vi "Actor Core.vi"(8 "error in":errorcluster, 11 "Panel Helper in":refnum<class "Panel Helper.lvclass">) -> (0 "error out":errorcluster, 3 "Actor out":refnum<class "Actor.lvclass">)   [LabVIEW 2020, in "2. Basic Panel Actors.lvlib" / "Panel Helper.lvclass"]
doc: "The user interface for this panel.\n----\nCopyright: MGI 2016\nAuthor: Derek Trepanier"
uses:
  Panel Helper.lvclass
  C:/Program Files/National Instruments/LabVIEW 2020/vi.lib/MGI/Panel Manager/Panel Actor/Panel Actor/Panel Actor.lvclass
  <vilib>/ActorFramework/Actor/Actor.lvclass
  <vilib>/ActorFramework/Message Enqueuer/Message Enqueuer.lvclass/Message Enqueuer.ctl
  <vilib>/MGI/Panel Manager/Panel/Panel Helper/Panel Helper.lvclass/Panel Helper.ctl
  <vilib>/ActorFramework/Message Enqueuer/Enqueue.vi
  Description Panel/Description Panel.lvclass
  <vilib>/MGI/Panel Manager/Panel/Panel/Subpanel/Subpanel.lvclass
  C:/Program Files/National Instruments/LabVIEW 2020/vi.lib/MGI/Panel Manager/Panel/Panel/Panel.lvclass
  <vilib>/ActorFramework/Stop Msg/Stop Msg.lvclass
  C:/Program Files/National Instruments/LabVIEW 2020/vi.lib/ActorFramework/Message/Message.lvclass
  <vilib>/MGI/Panel Manager/Panel/Panel/Subpanel/Subpanel.vi
  <vilib>/ActorFramework/Message Priority Queue/Priority Enqueue.vi
  <vilib>/MGI/Panel Manager/Panel/Deferer/Deferer.lvclass
  <vilib>/MGI/Panel Manager/Panel Actor/Panel Actor/Panel Actor.lvclass
  <vilib>/MGI/Panel Manager/Panel/Panel Updater/Panel Updater.lvclass
  <vilib>/MGI/Panel Manager/Panel/Panel.lvlib
  <vilib>/MGI/Panel Manager/Panel/Panel Helper/Panel Helper.lvclass
panel:
  in  "Clear Title":bool
  in  "Panel Title Override":string
  in  "Clear Tree":bool
  in  "Without Defer":bool
  in  "With Defer":bool
  in  "Tree":string(tree)
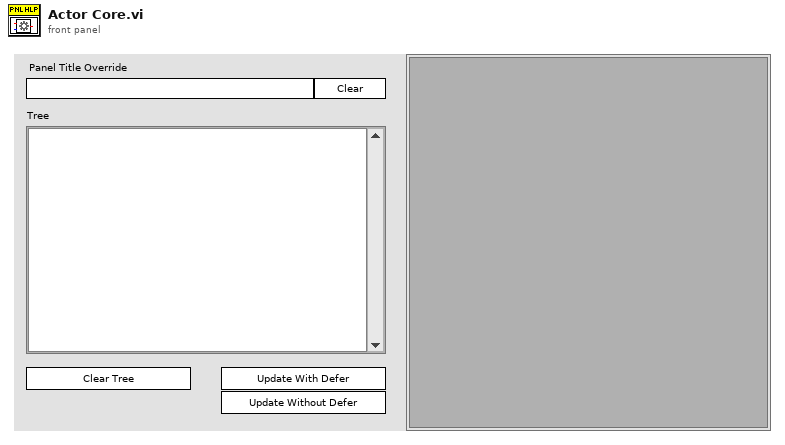
[diagram p1: front panel]
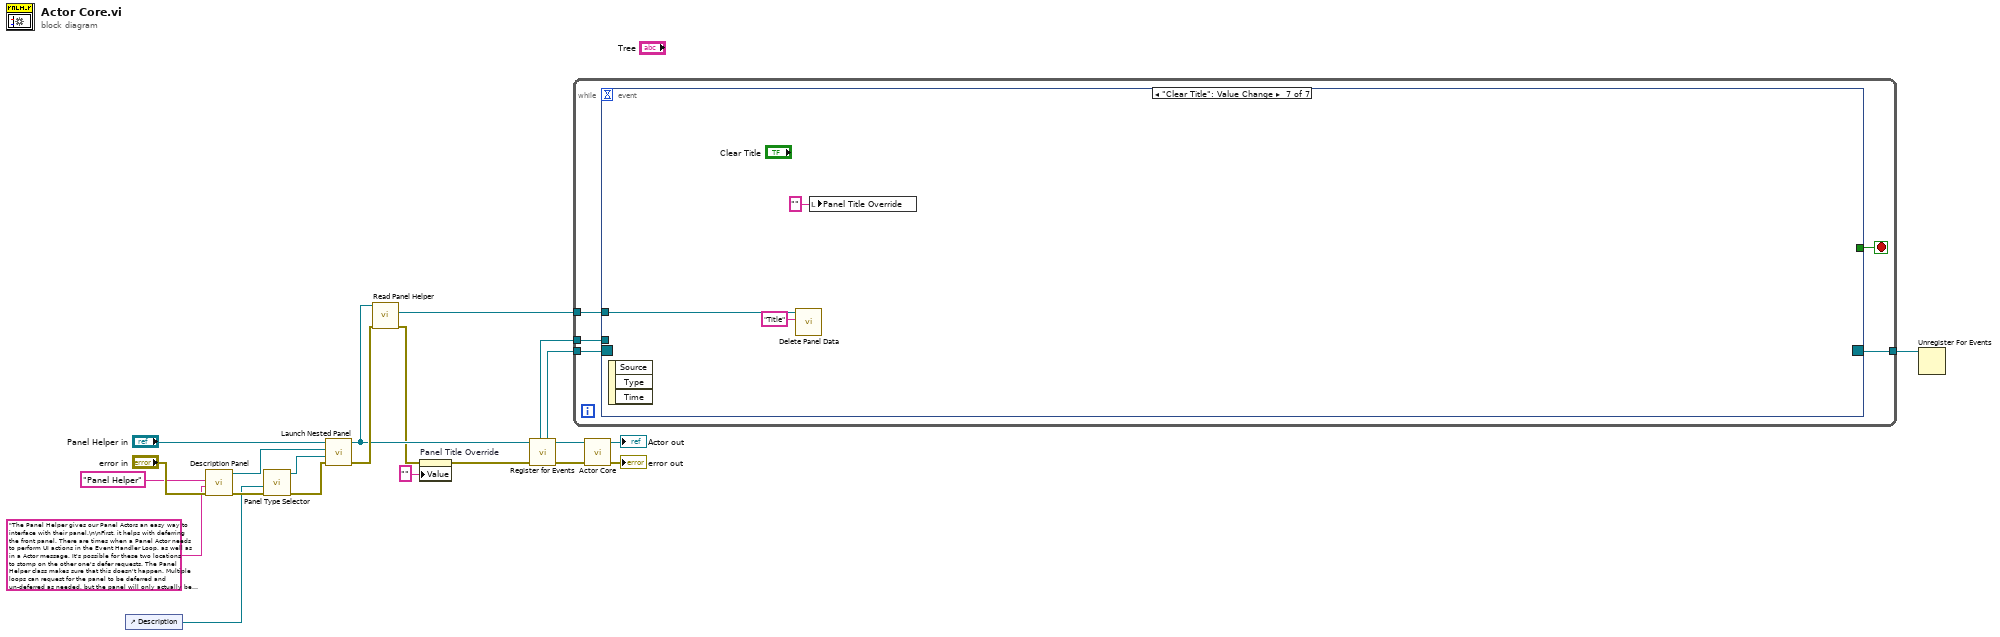
[diagram p0: block diagram]
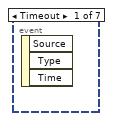
[diagram p2: hidden frame]
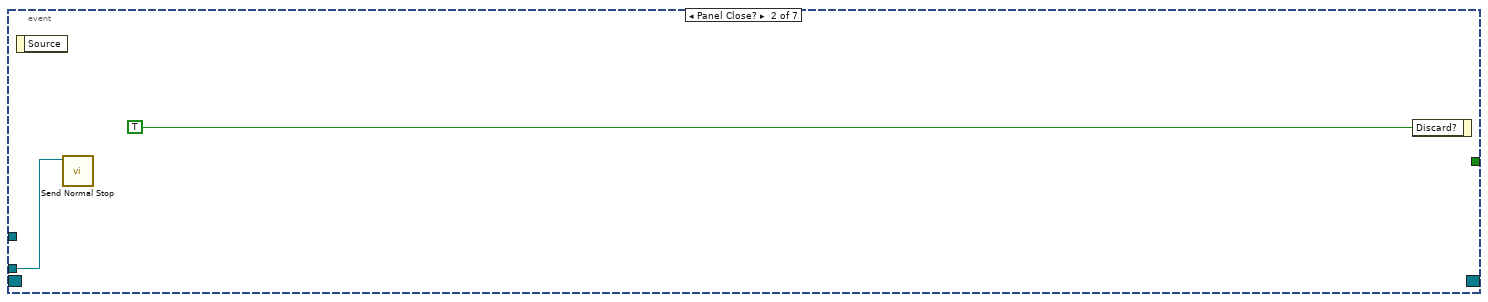
[diagram p3: hidden frame]
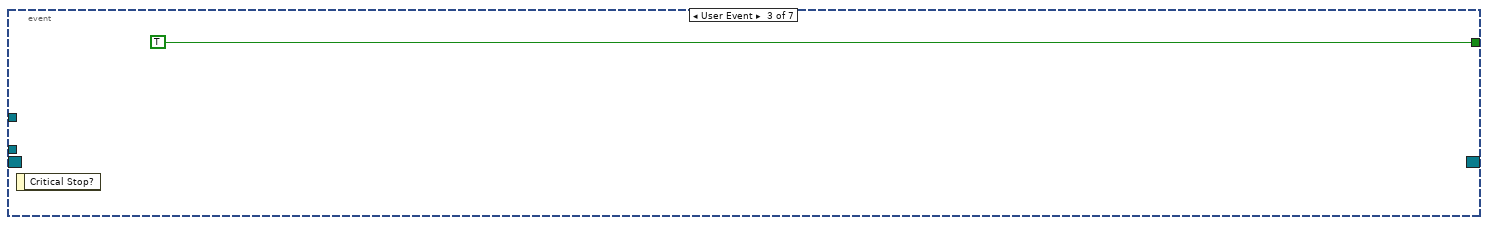
[diagram p4: hidden frame]
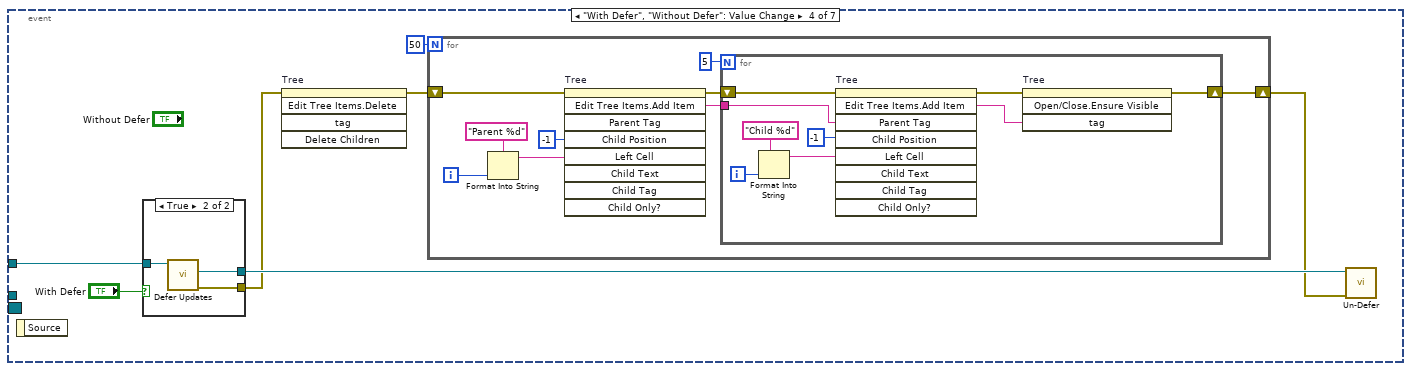
[diagram p5: hidden frame]
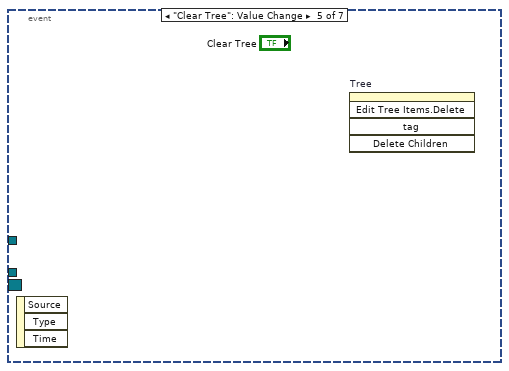
[diagram p7: hidden frame]
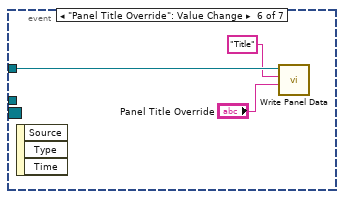
[diagram p8: hidden frame]
diagram:
  n1 = control-ref of="Description"() -> (w12:refnum<vi>)
  n2 = call "Description Panel.vi"("error in (no error)"="error in", "Description"="The Panel Helper gives our Panel Actors an easy way to interface with their panel.\n\nFirst, it helps with deferring the front panel. There are times when a Panel Actor needs to perform UI actions in the Event Handler Loop, as well as in a Actor message. It's possible for these two locations to stomp on the other one's defer requests. The Panel Helper class makes sure that this doesn't happen. Multiple loops can request for the panel to be deferred and un-deferred as needed, but the panel will only actually be un-deferred after all loops have un-deferred it.\n\nSecond, it manages the Panel Data. Panel Data gives the Panel Actor a way to interface with the active Panel object. Different Panel Classes use Panel Data differently so review the Panel Class's documentation for more info.\n\nThird, it manages the lifetime of several key framework references. There is a 1:1 relationship between an actual Front Panel, and a Panel Helper. This isn't true about Panel Classes. A Panel Actor can be running, and then receive a \"Change Panel\" message. The Panel object will then be closed, and a new Panel object will be opened. The Panel Helper object doesn't change though.\n\nThis example demonstrates how to use the deferrer using the tree control. Click the \"Update with Defer\" or \"Update Without Defer\" to see the difference.\n\nIt also demonstrates how to use the Panel Data to change the Panel's Title. The Window Panel Class uses the Panel Data Field \"Title\" to override the specified Panel's Title. So every time the Panel Data Field \"Title\" is updated, the Window Panel Object updates the Front Panel's Title. Different Panel Types use Panel Data differently. So if this Panel Actor was launched in a Subpanel for example, the Title field would be ignored. \n" ("Description Title"), "Description Title"="Panel Helper") -> ("error out"=w20:errorcluster, "Description Panel out"=w17:refnum<class "Description Panel.lvclass">)  [unwired: 7 in]
  n3 = call-poly <vilib>:"Panel Type Selector.vi"("Error In"=w20, "Sub Panel"=w12) -> ("Error Out"=w18:errorcluster, "Subpanel Out"=w19:refnum<class "Subpanel.lvclass">)  [unwired: 8 in]
  n4 = call <vilib>:"Launch Nested Panel.vi"("error in (no error)"=w18, "Panel"=w19, "Nested Panel Actor"=w17, "Panel Actor in"="Panel Helper in") -> ("error out"=w7:errorcluster, "Panel Actor out"=w5:refnum<class "Panel Helper.lvclass">)  [unwired: 4 in, 2 out]
  n5 = call <vilib>:"Read Panel Helper.vi"("Error In"=w7, "Panel Actor in"=w5) -> ("Error Out"=w3:errorcluster, "Panel Helper"=w6:refnum<class "Panel Helper.lvclass">)  [unwired: 8 in]
  n6 = property on="Panel Title Override" class="Str"(error in=w3, "Value"="" ("Panel Title Override")) -> (error out=w4:errorcluster)  [unwired: 1 in, 1 out]
  n7 = call <vilib>:"Register for Events.vi"("Error In"=w4, "Panel Actor in"=w5) -> ("Error Out"=w11:errorcluster, "Panel Actor out"=w10:refnum<class "Panel Helper.lvclass">, "Pnl Actor"=w9:refnum<event-registration>, "Self Enqueuer"=w8:refnum<class "Message Enqueuer.lvclass">)  [unwired: 6 in]
  n8 = while {
    tunnel: w9 -> [w27]
    tunnel: w8 -> [w26]
    tunnel: w6 -> [w24]
    tunnel: [w23] -> w1
    stop <- w25 stop-if-true
    n9 = event shown="[6] \"Clear Title\": Value Change" {
      selector: w27 -> [_ _ _ _ _ _ _]
      dyn-events: [_ _ _ _ _ _ _] -> w23
      timeout: _ -> [_ _ _ _ _ _ _]
      tunnel: w26 -> [_ w29 _ _ _ _ _]
      tunnel: [_ _ TRUE _ _ _ _] -> w25
      tunnel: w24 -> [_ _ _ w37 _ w61 w63]
      event Timeout {
        n10 = event-data() -> ()  [unwired: 1 in, 3 out]
      }
      event Panel Close? {
        n11 = event-data() -> ()  [unwired: 1 in, 1 out]
        n12 = call <vilib>:"Send Normal Stop.vi"("Message Enqueuer"=w29) -> ()  [unwired: 10 in, 1 out]
        n13 = event-data("Discard?"=TRUE) -> ()  [unwired: 1 in, 1 out]
      }
      event User Event {
        n14 = event-data() -> ()  [unwired: 1 in, 1 out]
      }
      event "With Defer", "Without Defer": Value Change {
        n15 = event-data() -> ()  [unwired: 1 in, 1 out]
        n16 = case shown="True" "With Defer" {
          tunnel: w37 -> [_ w58]
          tunnel: [_ w57] -> w36
          tunnel: [_ w56] -> w34
          frame False {
          }
          frame True {
            n17 = call <vilib>:"Defer Updates.vi"("Controller in"=w58) -> ("Error Out"=w56:errorcluster, "Deferer"=w57:refnum<class "Deferer.lvclass">)  [unwired: 9 in]
          }
        }
        n18 = invoke on="Tree" class="Tree (strict)" method="Edit Tree Items.Delete"(error in=w34) -> (error out=w33:errorcluster)  [unwired: 4 in, 4 out]
        n19 = for {
          N: 50 -> [_]
          shift-right: [w42] -> w31
          shift-left: w33 -> [w46]
          i -> [w44]
          n20 = Format Into String(format string="Parent %d", w44) -> (resulting string=w45:string)  [unwired: 2 in, 1 out]
          n21 = invoke on="Tree" class="Tree (strict)" method="Edit Tree Items.Add Item"(error in=w46, "Child Position"=-1, "Left Cell"=w45) -> (error out=w41:errorcluster, "Edit Tree Items:Add Item"=w39:string)  [unwired: 6 in, 7 out]
          n22 = for {
            N: 5 -> [_]
            shift-right: [w49] -> w42
            shift-left: w41 -> [w54]
            tunnel: w39 -> [w51]
            i -> [w53]
            n23 = Format Into String(format string="Child %d", w53) -> (resulting string=w52:string)  [unwired: 2 in, 1 out]
            n24 = invoke on="Tree" class="Tree (strict)" method="Edit Tree Items.Add Item"(error in=w54, "Parent Tag"=w51, "Child Position"=-1, "Left Cell"=w52) -> (error out=w50:errorcluster, "Edit Tree Items:Add Item"=w48:string)  [unwired: 5 in, 7 out]
            n25 = invoke on="Tree" class="Tree (strict)" method="Open/Close.Ensure Visible"(error in=w50, "tag"=w48) -> (error out=w49:errorcluster)  [unwired: 2 in, 3 out]
          }
        }
        n26 = call <vilib>:"Un-Defer.vi"("Error In"=w31, "Deferer in"=w36) -> ()  [unwired: 9 in, 1 out]
      }
      event "Clear Tree": Value Change {
        n27 = event-data() -> ()  [unwired: 1 in, 3 out]
        n28 = invoke on="Tree" class="Tree (strict)" method="Edit Tree Items.Delete"() -> ()  [unwired: 5 in, 5 out]
      }
      event "Panel Title Override": Value Change {
        n29 = event-data() -> ()  [unwired: 1 in, 3 out]
        n30 = call <vilib>:"Write Panel Data.vi"("Panel Data"="Panel Title Override", "Field"="Title", "Panel Helper in"=w61) -> ()  [unwired: 7 in, 2 out]
      }
      event "Clear Title": Value Change {
        n31 = event-data() -> ()  [unwired: 1 in, 3 out]
        n32 = call <vilib>:"Delete Panel Data.vi"("Field"="Title", "Panel Helper in"=w63) -> ()  [unwired: 8 in, 2 out]
        n33 = local write "Panel Title Override"("" ("Panel Title Override")) -> ()
      }
    }
  }
  n34 = call-parent "Actor Core.vi"("error in"=w11, "Panel Actor in"=w10) -> ("error out"=→"error out":errorcluster, "Actor out"=→"Actor out":refnum<class "Actor.lvclass">)  [unwired: 8 in]
  n35 = Unregister For Events(event registration refnum=w1) -> ()  [unwired: 1 in, 1 out]
